vi "BB_SendAnglesDistanceTime.vi"(11 "Cluster":T1) -> ()   [LabVIEW 2012]
uses:
  typeDefs/targetVariables.ctl
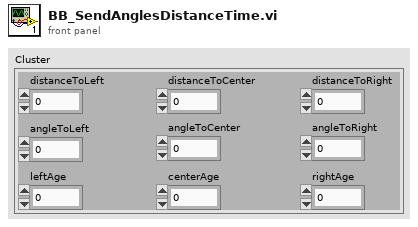
[diagram p1: front panel]
types:
  T1 = typedef "targetVariables.ctl" = cluster{"distanceToCenter":dbl, "angleToCenter":dbl, "angleToLeft":dbl, "distanceToLeft":dbl, "angleToRight":dbl, "distanceToRight":dbl, "centerAge":dbl, "leftAge":dbl, "rightAge":dbl}
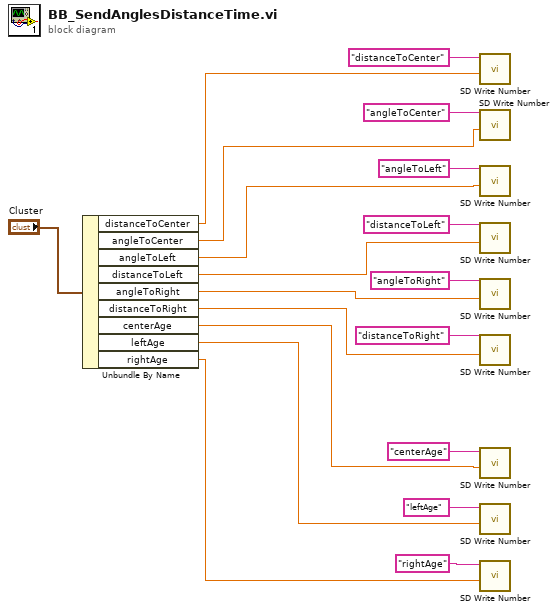
[diagram p0: block diagram]
diagram:
  n1 = Unbundle By Name("Cluster") -> ("distanceToCenter"=w9:dbl, "angleToCenter"=w8:dbl, "angleToLeft"=w7:dbl, "distanceToLeft"=w6:dbl, "angleToRight"=w5:dbl, "distanceToRight"=w4:dbl, "centerAge"=w3:dbl, "leftAge"=w2:dbl, "rightAge"=w1:dbl)
  n2 = call <vilib>:"SD Write Number.vi"("Numeric"=w9, "Name"="distanceToCenter") -> ()  [unwired: 8 in, 2 out]
  n3 = call <vilib>:"SD Write Number.vi"("Numeric"=w8, "Name"="angleToCenter") -> ()  [unwired: 8 in, 2 out]
  n4 = call <vilib>:"SD Write Number.vi"("Numeric"=w7, "Name"="angleToLeft") -> ()  [unwired: 8 in, 2 out]
  n5 = call <vilib>:"SD Write Number.vi"("Numeric"=w6, "Name"="distanceToLeft") -> ()  [unwired: 8 in, 2 out]
  n6 = call <vilib>:"SD Write Number.vi"("Numeric"=w5, "Name"="angleToRight") -> ()  [unwired: 8 in, 2 out]
  n7 = call <vilib>:"SD Write Number.vi"("Numeric"=w4, "Name"="distanceToRight") -> ()  [unwired: 8 in, 2 out]
  n8 = call <vilib>:"SD Write Number.vi"("Numeric"=w3, "Name"="centerAge") -> ()  [unwired: 8 in, 2 out]
  n9 = call <vilib>:"SD Write Number.vi"("Numeric"=w2, "Name"="leftAge") -> ()  [unwired: 8 in, 2 out]
  n10 = call <vilib>:"SD Write Number.vi"("Numeric"=w1, "Name"="rightAge") -> ()  [unwired: 8 in, 2 out]
